vi "Generator VI.vi"() -> ()   [LabVIEW 2010]
doc: "This VI in conjunction with Display VI.vi demonstrates how to use network streams to pass data and commands between two running VIs. It generates waveforms of the specified type and updates the type of waveform as it receives commands from the Display VI.\n\n<B>Note:</B> Requires Display VI.vi located in the same directory as this VI."
uses:
  <vilib>/measure/NI_MABase.lvlib
panel:
  in  "Stop":bool
  out "Command":string
  out "error oout":errorcluster
  # "Instructions:\n1. Open the Display VI.vi located in the same directory.\n2. Follow the instructions on its front panel."
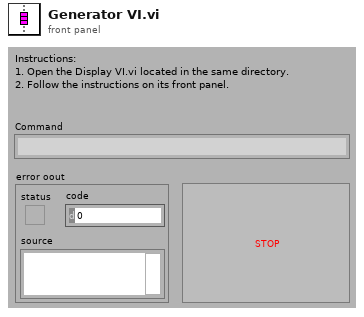
[diagram p1: front panel]
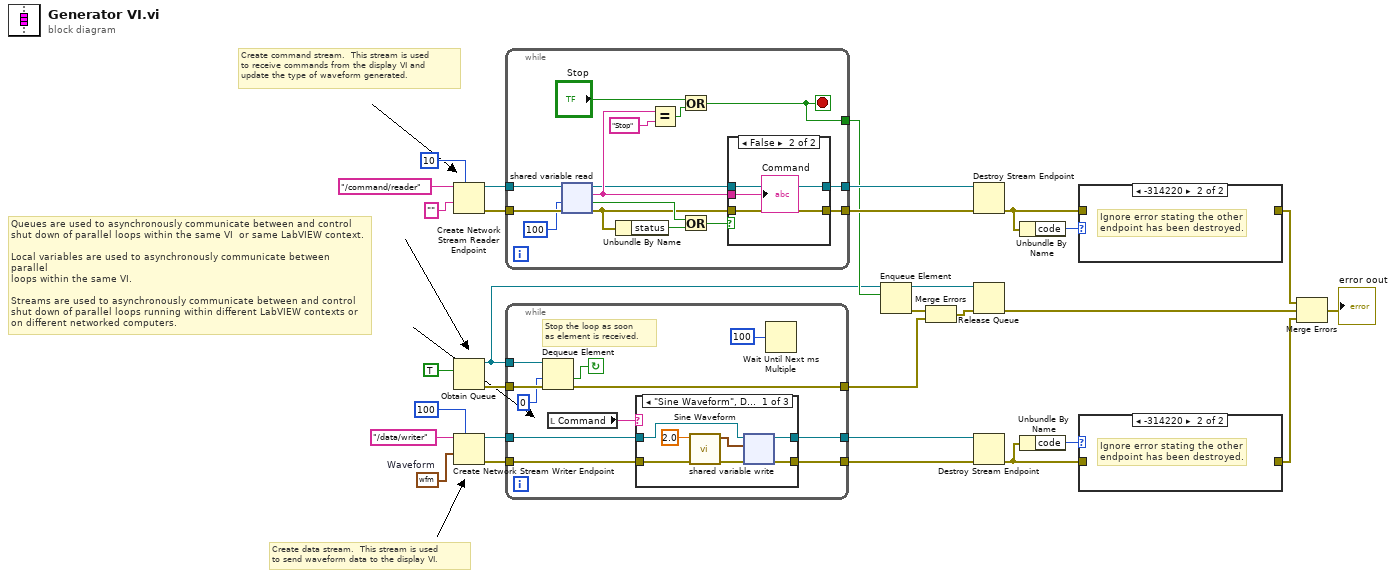
[diagram p0: block diagram]
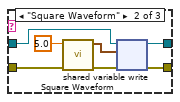
[diagram p4: hidden frame]
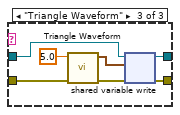
[diagram p5: hidden frame]
diagram:
  w21 = waveform(dbl) {"t0"=timestamp(0 s since 1904-01-01), "dt"=1.0, "Y"=[]}  # Waveform
  # "Queues are used to asynchronously communicate between and control \nshut down of parallel loops within the same VI  or same LabVIEW context.  \n\nLocal variables are used to asynchronously communicate between parallel\nloops within the same VI.\n\nStreams are used to asynchronously communicate between and control \nshut down of parallel loops running within different LabVIEW contexts or \non different networked computers."
  # "Create data stream.  This stream is used\nto send waveform data to the display VI."
  # "Create command stream.  This stream is used\nto receive commands from the display VI and \nupdate the type of waveform generated."
  n1 = Create Network Stream Reader Endpoint(7:10 ("reader buffer size"), 9:"", 11:"/command/reader" ("reader name")) -> (0:w27:errorcluster, 3:w28:refnum<k21>)  [unwired: 3 in]
  n2 = Obtain Queue(element data type=TRUE ("stop")) -> (queue out=w10:refnum<queue>, error out=w17:errorcluster)  [unwired: 4 in, 1 out]
  n3 = Create Network Stream Writer Endpoint(7:100 ("writer buffer size"), 9:w21, 11:"/data/writer" ("writer name")) -> (0:w22:errorcluster, 3:w23:refnum<k21>)  [unwired: 3 in]
  n4 = while {
    tunnel: w28 -> [w45]
    tunnel: w27 -> [w44]
    tunnel: [w37] -> w26
    tunnel: [w31] -> w25
    tunnel: [w39] -> w11
    stop <- w39 stop-if-true
    n5 = shared-variable-read(w45, w44, 100 ("timeout ms")) -> (w32:refnum<k21>, w38:errorcluster, w41:bool, w34:string)
    n6 = Unbundle By Name(w38) -> ("status"=w42:bool)
    n7 = Equal?(x=w34, y="Stop" ("x")) -> (x = y?=w35:bool)
    n8 = Or(x="Stop", y=w35) -> (x .or. y?=w39:bool)
    n9 = Or(x=w41, y=w42) -> (x .or. y?=w40:bool)
    n10 = case shown="False" w40 {
      tunnel: w34 -> [_ w50]
      tunnel: w38 -> [w47 w49]
      tunnel: [w47 w49] -> w37
      tunnel: w32 -> [w46 w48]
      tunnel: [w46 w48] -> w31
      frame True {
      }
      frame False {
        "Command" <- w50
      }
    }
  }
  n11 = while {
    tunnel: w23 -> [w60]
    tunnel: w22 -> [w59]
    tunnel: [w58] -> w20
    tunnel: [w57] -> w19
    tunnel: w17 -> [w55]
    tunnel: w10 -> [w54]
    tunnel: [w51] -> w1
    stop <- w52 continue-if-true
    # "Stop the loop as soon \nas element is received."
    n12 = Dequeue Element(queue=w54, timeout in ms (-1)=0, error in (no error)=w55) -> (timed out?=w52:bool, error out=w51:errorcluster)  [unwired: 2 out]
    n13 = local read "Command"() -> (w61:string)
    n14 = case shown="\"Sine Waveform\", Default" w61 {
      tunnel: w60 -> [w67 w74 w81]
      tunnel: w59 -> [w66 w73 w80]
      tunnel: [w64 w71 w78] -> w58
      tunnel: [w63 w70 w77] -> w57
      frame "Sine Waveform", Default {
        n15 = call <vilib>:"Sine Waveform.vi"("error in (no error)"=w66, "frequency"=2.0) -> ("error out"=w68:errorcluster, "signal out"=w65:waveform(dbl))  [unwired: 8 in]
        n16 = shared-variable-write(w67, w68, w65) -> (w63:refnum<k21>, w64:errorcluster)  [unwired: 1 in, 1 out]
      }
      frame "Square Waveform" {
        n17 = call <vilib>:"Square Waveform.vi"("error in (no error)"=w73, "frequency"=5.0) -> ("error out"=w75:errorcluster, "signal out"=w72:waveform(dbl))  [unwired: 8 in]
        n18 = shared-variable-write(w74, w75, w72) -> (w70:refnum<k21>, w71:errorcluster)  [unwired: 1 in, 1 out]
      }
      frame "Triangle Waveform" {
        n19 = call <vilib>:"Triangle Waveform.vi"("error in (no error)"=w80, "frequency"=5.0) -> ("error out"=w82:errorcluster, "signal out"=w79:waveform(dbl))  [unwired: 8 in]
        n20 = shared-variable-write(w81, w82, w79) -> (w77:refnum<k21>, w78:errorcluster)  [unwired: 1 in, 1 out]
      }
    }
    n21 = Wait Until Next ms Multiple(millisecond multiple=u32 100 ("milliseconds to wait")) -> ()  [unwired: 1 out]
  }
  n22 = Enqueue Element(queue=w10, element=w11) -> (queue out=w14:refnum<queue>, error out=w13:errorcluster)  [unwired: 2 in, 1 out]
  n23 = Merge Errors(w13, w1) -> (w12:errorcluster)
  n24 = Destroy Stream Endpoint(8:w26, 11:w25) -> (0:w8:errorcluster)
  n25 = Release Queue(queue=w14, error in (no error)=w12) -> (error out=w5:errorcluster)  [unwired: 1 in, 2 out]
  n26 = Destroy Stream Endpoint(8:w20, 11:w19) -> (0:w6:errorcluster)
  n27 = Unbundle By Name(w8) -> ("code"=w9:i32)
  n28 = Unbundle By Name(w6) -> ("code"=w7:i32)
  n29 = case shown="-314220" w9 {
    tunnel: w8 -> [w83 _]
    tunnel: [w83 _] -> w3
    frame 0, Default {
    }
    frame -314220 {
      # "Ignore error stating the other\nendpoint has been destroyed."
    }
  }
  n30 = case shown="-314220" w7 {
    tunnel: w6 -> [w84 _]
    tunnel: [w84 _] -> w4
    frame 0, Default {
    }
    frame -314220 {
      # "Ignore error stating the other\nendpoint has been destroyed."
    }
  }
  n31 = Merge Errors(w3, w5, w4) -> (→"error oout":errorcluster)
